vi "Wait for Loop Synch.vi"(8 "Error In":errorcluster) -> (0 "Error Out":errorcluster)   [LabVIEW 2014]
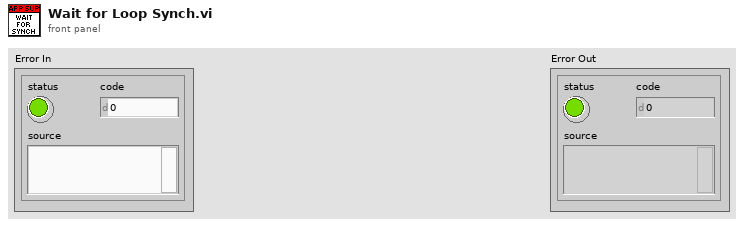
[diagram p1: front panel]
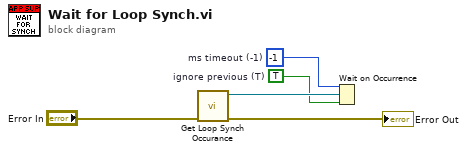
[diagram p0: block diagram]
diagram:
  w3 = -1  # ms timeout (-1)
  w4 = TRUE  # ignore previous (T)
  n1 = call "Get Loop Synch Occurance.vi"("Error In"="Error In") -> ("Error Out"=→"Error Out":errorcluster, "Loop Synch Occourance"=w5:refnum<k4>)  [unwired: 9 in]
  n2 = Wait on Occurrence(1:w4, 2:w5, 3:w3) -> ()  [unwired: 1 out]
